vi "RW_Mutex_Take.vi"(10 "error in (no error)":errorcluster) -> (2 "error out":errorcluster)   [LabVIEW 2016]
uses:
  RW_Mutex.vi
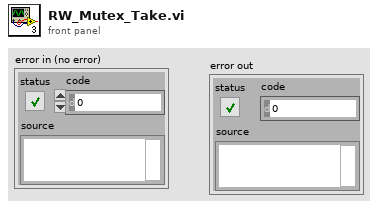
[diagram p1: front panel]
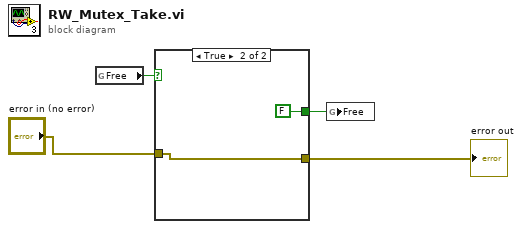
[diagram p0: block diagram]
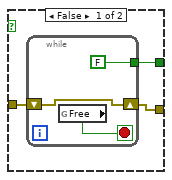
[diagram p2: hidden frame]
diagram:
  n1 = global read "RW_Mutex.vi" "Free"() -> (w4:bool)
  n2 = case shown="True" w4 {
    tunnel: [w7 FALSE] -> w3
    tunnel: "error in (no error)" -> [w6 w11]
    tunnel: [w5 w11] -> w1
    frame False {
      n3 = while {
        tunnel: [FALSE] -> w7
        shift-right: [w8] -> w5
        shift-left: w6 -> [w8]
        stop <- w10 stop-if-true
        n4 = global read "RW_Mutex.vi" "Free"() -> (w10:bool)
      }
    }
    frame True {
    }
  }
  "error out" <- w1
  n5 = global write "RW_Mutex.vi" "Free"(w3) -> ()
